vi "Add Labels in Setup Group.vi"(0 "engine in":refnum<k7>, 5 "sequence file in":refnum<k7>, 11 "error in":errorcluster) -> (4 "engine out":refnum<k7>, 6 "sequence file out":refnum<k7>, 15 "error out":errorcluster)   [LabVIEW 2021, in "Create Sequence.lvlib"]
doc: "Adds the required instruction steps on the 'SetupGroup'"
uses:
  Create Sequence.lvlib
  TypeDef/Step Properties.ctl
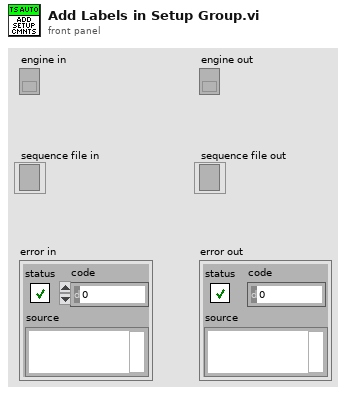
[diagram p1: front panel]
types:
  T1 = typedef "Create Sequence.lvlib/Step Properties.ctl" = cluster{"step type name":string, "step name":string, "description":string, "comment":string, "sequence name param":string, "step group":i32, "step index":i32, "expression":string}
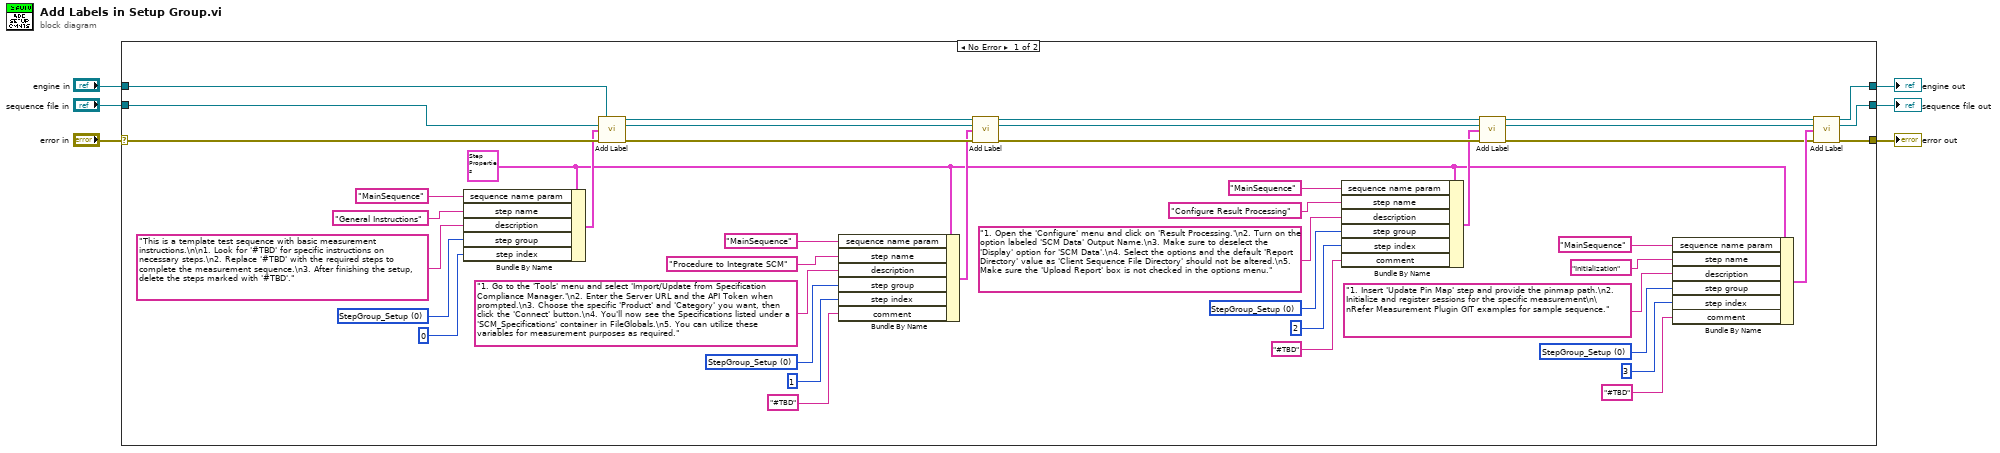
[diagram p0: block diagram]
diagram:
  n1 = case shown="No Error" "error in" {
    selector: "error in" -> [w43 w52]
    tunnel: "engine in" -> [w39 w50]
    tunnel: "sequence file in" -> [w41 w51]
    tunnel: [w46 w50] -> w3
    tunnel: [w45 w51] -> w2
    tunnel: [w44 w52] -> w1
    frame No Error {
      w17 = 0 items=["StepGroup_Setup", "StepGroup_Main", "StepGroup_Cleanup"] ("Step Group")
      w25 = 0 items=["StepGroup_Setup", "StepGroup_Main", "StepGroup_Cleanup"] ("Step Group")
      w28 = 0 items=["StepGroup_Setup", "StepGroup_Main", "StepGroup_Cleanup"] ("Step Group")
      w15 = T1 {"step type name"="", "step name"="", "description"="", "comment"="", "sequence name param"="MainSequence", "step group"=0, "step index"=3, "expression"=""} ("StepProperties")
      w35 = 0 items=["StepGroup_Setup", "StepGroup_Main", "StepGroup_Cleanup"] ("Step Group")
      n2 = Bundle By Name(cluster=w15, "sequence name param"="MainSequence" ("sequenceNameParam"), "step name"="General Instructions" ("Step Name"), "description"="This is a template test sequence with basic measurement instructions.\n\n1. Look for '#TBD' for specific instructions on necessary steps.\n2. Replace '#TBD' with the required steps to complete the measurement sequence.\n3. After finishing the setup, delete the steps marked with '#TBD'." ("Description"), "step group"=w35, "step index"=0 ("Step Index")) -> (w33:T1)
      n3 = call "Add Label.vi"("engine in"=w39, "sequence file in"=w41, "step properties"=w33, "error in"=w43) -> ("engine out"=w38:refnum<k7>, "sequence file out"=w40:refnum<k7>, "error out"=w42:errorcluster)  [unwired: 9 in]
      n4 = Bundle By Name(cluster=w15, "sequence name param"="MainSequence" ("sequenceNameParam"), "step name"="Procedure to Integrate SCM" ("Step Name"), "description"="1. Go to the 'Tools' menu and select 'Import/Update from Specification Compliance Manager.'\n2. Enter the Server URL and the API Token when prompted.\n3. Choose the specific 'Product' and 'Category' you want, then click the 'Connect' button.\n4. You'll now see the Specifications listed under a 'SCM_Specifications' container in FileGlobals.\n5. You can utilize these variables for measurement purposes as required." ("Description"), "step group"=w28, "step index"=1 ("Step Index"), "comment"="#TBD" ("Comment")) -> (w32:T1)
      n5 = call "Add Label.vi"("engine in"=w38, "sequence file in"=w40, "step properties"=w32, "error in"=w42) -> ("engine out"=w47:refnum<k7>, "sequence file out"=w48:refnum<k7>, "error out"=w49:errorcluster)  [unwired: 9 in]
      n6 = Bundle By Name(cluster=w15, "sequence name param"="MainSequence" ("sequenceNameParam"), "step name"="Configure Result Processing" ("Step Name"), "description"="1. Open the 'Configure' menu and click on 'Result Processing.'\n2. Turn on the option labeled 'SCM Data' Output Name.\n3. Make sure to deselect the 'Display' option for 'SCM Data'.\n4. Select the options and the default 'Report Directory' value as 'Client Sequence File Directory' should not be altered.\n5. Make sure the 'Upload Report' box is not checked in the options menu." ("Description"), "step group"=w25, "step index"=2 ("Step Index"), "comment"="#TBD" ("Comment")) -> (w21:T1)
      n7 = call "Add Label.vi"("engine in"=w47, "sequence file in"=w48, "step properties"=w21, "error in"=w49) -> ("engine out"=w13:refnum<k7>, "sequence file out"=w12:refnum<k7>, "error out"=w11:errorcluster)  [unwired: 9 in]
      n8 = Bundle By Name(cluster=w15, "sequence name param"="MainSequence" ("sequenceNameParam"), "step name"="Initialization" ("Step Name"), "description"="1. Insert 'Update Pin Map' step and provide the pinmap path.\n2. Initialize and register sessions for the specific measurement\n\nRefer Measurement Plugin GIT examples for sample sequence." ("Description"), "step group"=w17, "step index"=3 ("Step Index"), "comment"="#TBD" ("Comment")) -> (w14:T1)
      n9 = call "Add Label.vi"("engine in"=w13, "sequence file in"=w12, "step properties"=w14, "error in"=w11) -> ("engine out"=w46:refnum<k7>, "sequence file out"=w45:refnum<k7>, "error out"=w44:errorcluster)  [unwired: 9 in]
    }
    frame Error {
    }
  }
  "error out" <- w1
  "engine out" <- w3
  "sequence file out" <- w2
